vi "get Text Size.vi"(10 "Text":string, 11 "Font Pointer":u32 format="%.0x") -> (2 "Height":i32, 3 "Width":i32)   [LabVIEW 2015, in "LibSDL2_TTF.lvlib"]
uses:
  LibSDL2_TTF.lvlib
  LibSDL2 Wrapper/DLL/SDL2_ttf.dll
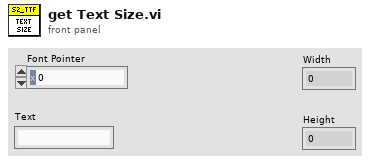
[diagram p1: front panel]
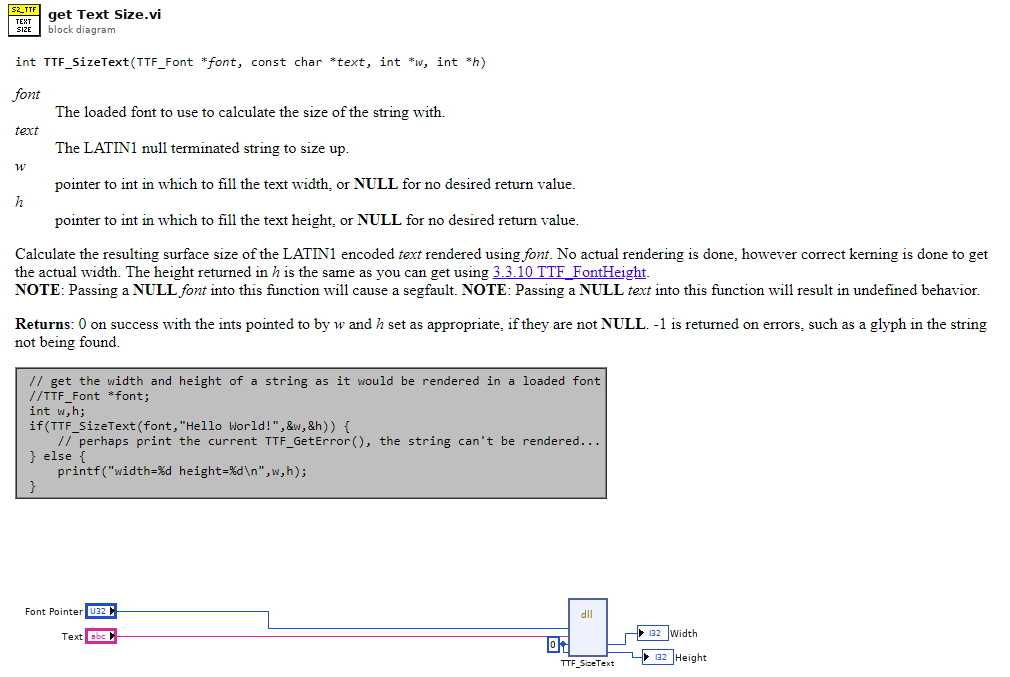
[diagram p0: block diagram]
diagram:
  w3 = 0 ("Width")
  n1 = dll-call lib="C:/dev/PGS/LabSDL2/Source/Libraries/LibSDL2 Wrapper/DLL/SDL2_ttf.dll" fn="TTF_SizeText"("Font Pointer"="Font Pointer", "Text"="Text", "Width"=w3, "Height"=w3) -> ("Width"=→"Width":i32, "Height"=→"Height":i32)  [unwired: 6 in, 2 out]
